vi "Create Map from Port-Label-SDI to Channel Index.vi"(11 "RT hardware channel data":T2[](array[typedef]) {"labels settings for RT"."Label Timestamp Channel Data Reference" format="%.0x"; "labels settings for RT"."Word Initial Raw Value" format="%032.0f"; "labels settings for RT"."Label Disable/Trigger Channel Reference" format="%.0x"; "labels settings for RT"."parameter driver data"."Tx parameter refs" format="%.0x"; "labels settings for RT"."parameter driver data"."Rx block data refs"."Data Reference" format="%.0x"; "labels settings for RT"."SDI" format="%02b"; "labels settings for RT"."label" format="%.0o"}) -> ()   [LabVIEW 2020, in "Ballard ARINC 429 Engine.lvlib" / "Custom Device.lvlib"]
uses:
  Custom Device.lvlib
  Shared/RT Hardware Channel Settings.ctl
  Shared/RT Label Settings.ctl
  Shared/Label.ctl
  Shared/RT Parameters.ctl
  Shared/Parameter Definition.ctl
  Encoding and Decoding/Encoding.ctl
  <vilib>/NI VeriStand/Custom Device API/Block Data Reference.ctl
  <vilib>/NI VeriStand/Custom Device API/Data Reference.ctl
  <vilib>/NI VeriStand/Custom Device API/Custom Device Item Ref.ctl
  Shared/Transfer Type.ctl
  Shared/Map of Identifiers to Indexes.ctl
  Encoding and Decoding/Encoding and Decoding.lvlib
  <vilib>/NI VeriStand/Custom Device API/Custom Device API.lvlib
panel:
  out "Map":T1
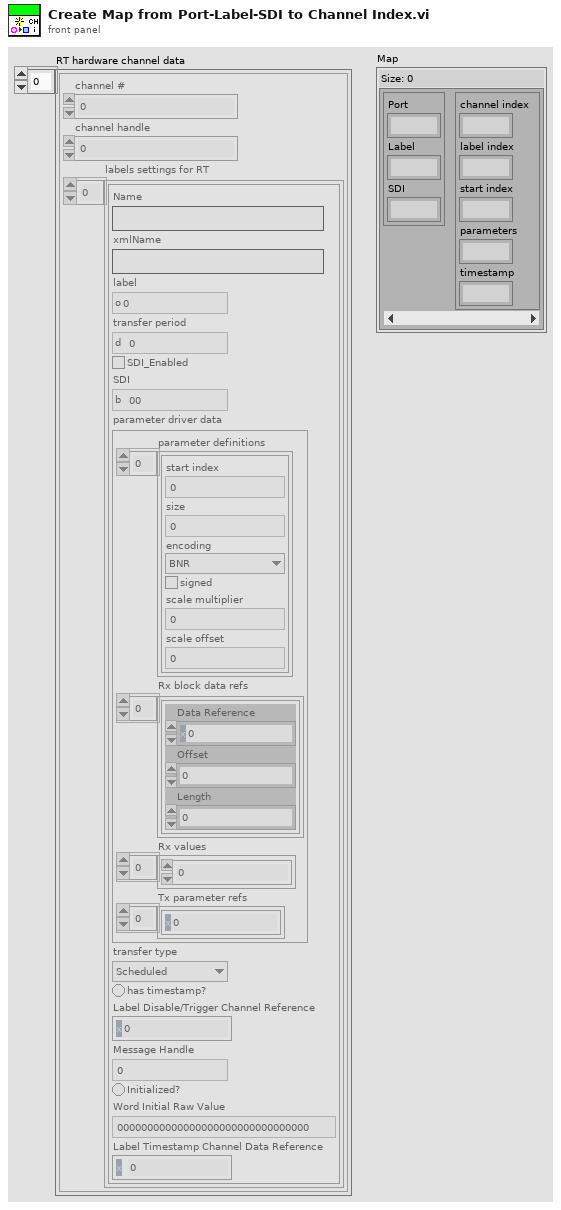
[diagram p1: front panel]
types:
  T1 = typedef "Map of Identifiers to Indexes.ctl" = map{cluster{"Port":u8, "Label":u8, "SDI":u8}, cluster{"channel index":i32, "label index":i32, "start index":i32, "parameters":i32, "timestamp":i32}}
  T2 = typedef "RT Hardware Channel Settings.ctl" = cluster{"channel #":u16, "channel handle":u64, "labels settings for RT":T3[]}
  T3 = typedef "RT Label Settings.ctl" = cluster{"Name":string, "xmlName":string, "label":T4, "transfer period":u32, "SDI_Enabled":bool, "SDI":u8, "parameter driver data":T5, "transfer type":T11, "has timestamp?":bool, "Label Disable/Trigger Channel Reference":T10, "Message Handle":u64, "Initialized?":bool, "Word Initial Raw Value":u32, "Label Timestamp Channel Data Reference":T9}
  T4 = typedef "Label.ctl" = u8
  T5 = typedef "RT Parameters.ctl" = cluster{"parameter definitions":T6[], "Rx block data refs":T8[], "Rx values":dbl[], "Tx parameter refs":T10[]}
  T6 = typedef "Parameter Definition.ctl" = cluster{"start index":i32, "size":i32, "encoding":T7, "signed":bool, "scale multiplier":dbl, "scale offset":dbl}
  T7 = typedef "Encoding and Decoding.lvlib/Encoding.ctl" = enum16{"BNR", "BCD", "Discrete"}
  T8 = typedef "Custom Device API.lvlib/Block Data Reference.ctl" = cluster{"Data Reference":T9, "Offset":u64, "Length":u64}
  T9 = typedef "Custom Device API.lvlib/Data Reference.ctl" = i32
  T10 = typedef "Custom Device API.lvlib/Custom Device Item Ref.ctl" = u64
  T11 = typedef "Transfer Type.ctl" = enum16{"Scheduled", "Acyclic", "Block", "Strobe"}
  T12 = cluster{"channel index":i32, "label index":i32, "start index":i32, "parameters":i32, "timestamp":i32}
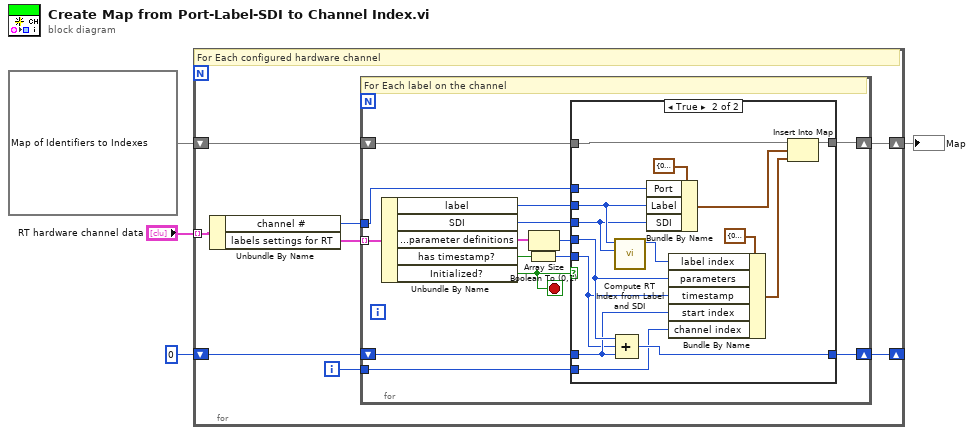
[diagram p0: block diagram]
diagram:
  n1 = for {
    tunnel: "RT hardware channel data" -> [w12] mode=indexing
    shift-right: [w7] -> w1
    shift-left: T1 {} -> [w9]
    shift-right: [w6] -> _
    shift-left: 0 -> [w8]
    i -> [w5]
    # "For Each configured hardware channel"
    n2 = Unbundle By Name(w12) -> ("channel #"=w10:u16, "labels settings for RT"=w11:T3[])
    n3 = for {
      tunnel: w11 -> [w24] mode=indexing
      tunnel: w10 -> [w22]
      shift-right: [w15] -> w7
      shift-left: w9 -> [w18]
      shift-right: [w16] -> w6
      shift-left: w8 -> [w21]
      tunnel: w5 -> [w13]
      stop <- w14 stop-if-true
      # "For Each label on the channel"
      n4 = Unbundle By Name(w24) -> ("label"=w23:T4, "SDI"=w17:u8, "parameter driver data.parameter definitions"=w26:T6[], "has timestamp?"=w25:bool, "Initialized?"=w14:bool)
      n5 = Boolean To (0,1)(Boolean=w25) -> (0, 1=w19:i16)
      n6 = Array Size(array=w26) -> (size(s)=w20:i32)
      n7 = case shown="True" w14 {
        tunnel: w23 -> [_ w32]
        tunnel: w22 -> [_ w42]
        tunnel: w21 -> [w27 w37]
        tunnel: w20 -> [_ w39]
        tunnel: w19 -> [_ w36]
        tunnel: w18 -> [w28 w43]
        tunnel: w17 -> [_ w31]
        tunnel: [w27 w38] -> w16
        tunnel: [w28 w35] -> w15
        tunnel: w13 -> [_ w29]
        frame False {
        }
        frame True {
          n8 = call "Compute RT Index from Label and SDI.vi"("SDI"=w31, "label"=w32) -> ("RT label index"=w30:i32)  [unwired: 9 in]
          n9 = Compound Arithmetic op=ADD(w39, w36, w37) -> (w38:i32)
          n10 = Bundle By Name(cluster=cluster{"Port":u8, "Label":u8, "SDI":u8} {"Port"=0, "Label"=0, "SDI"=0} ("key"), "Port"=w42, "Label"=w32, "SDI"=w31) -> (w40:cluster{"Port":u8, "Label":u8, "SDI":u8})
          n11 = Bundle By Name(cluster=T12 {"channel index"=0, "label index"=0, "start index"=0, "parameters"=0, "timestamp"=0} ("value"), "label index"=w30, "parameters"=w39, "timestamp"=w36, "start index"=w37, "channel index"=w29) -> (w33:T12)
          n12 = Insert Into Map(map in=w43, key=w40, value=w33) -> (map out=w35:T1)  [unwired: 2 out]
        }
      }
    }
  }
  "Map" <- w1
